vi "rename tag writer or reader.vi"(6 "new channel":refnum<class "TBM channel.lvclass">, 7 "owner ID":string, 8 "error in":errorcluster, 9 "old channel":refnum<class "TBM channel.lvclass">, 10 "tag descriptor":refnum<class "tag descriptor.lvclass">, 11 "engine configuration in":refnum<class "engine configuration.lvclass">) -> (0 "error out":errorcluster, 3 "engine configuration out":refnum<class "engine configuration.lvclass">)   [LabVIEW 2013, in "engine configuration.lvclass"]
uses:
  engine configuration.lvclass
  <vilib>/NI/Tag Bus/tag/tag descriptor.lvclass
  <vilib>/NI/Tag Bus Module Framework/channel/TBM channel.lvclass
  <vilib>/NI/Tag Bus/tag/tag descriptor.lvclass/tag descriptor.ctl
  engine configuration.lvclass/engine configuration.ctl
  <vilib>/NI/Tag Bus Module Framework/channel/TBM channel.lvclass/TBM channel.ctl
  <vilib>/NI/Tag Bus/tag/read tag name.vi
  <vilib>/NI/Tag Bus Module Framework/channel/Read channel classification.vi
  <vilib>/NI/Tag Bus Module Framework/root configuration/TBM configuration.lvclass
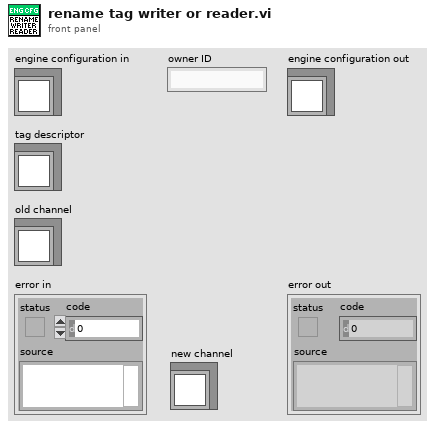
[diagram p1: front panel]
types:
  T1 = typedef "engine configuration.lvclass/Tag Info.ctl" = cluster{"Tag":refnum<class "tag descriptor.lvclass">, "Writer":string, "Readers":string[], "Owning ID":string}
  T2 = typedef "TBM channel.lvclass/channel classification.ctl" = enum16{"input data", "output data", "processing parameter", "processing result"}
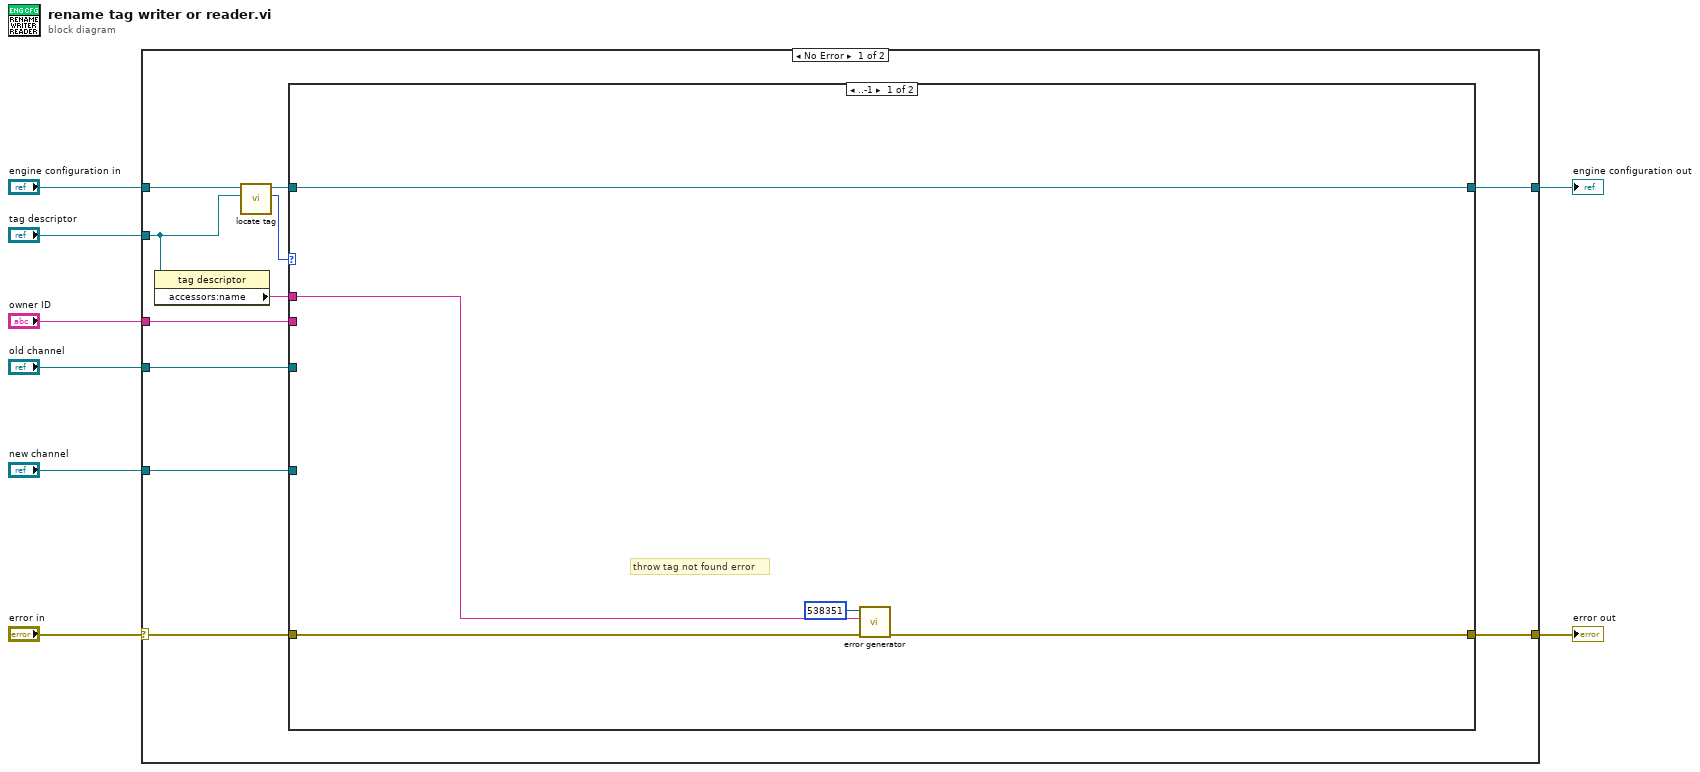
[diagram p0: block diagram]
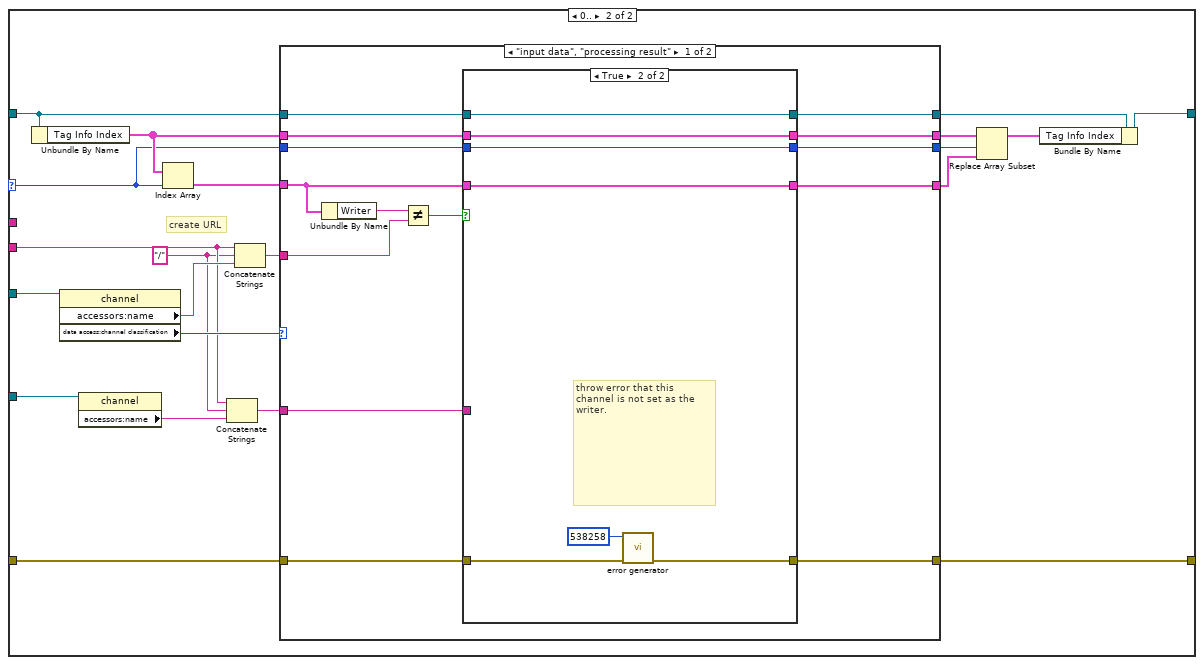
[diagram p2: hidden frame]
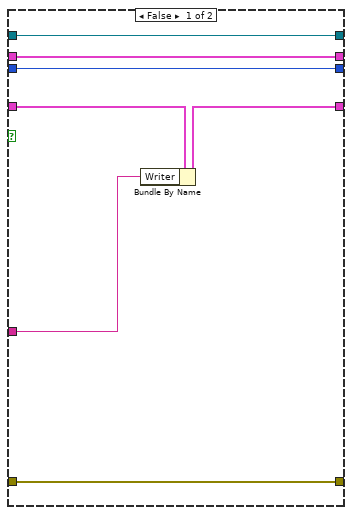
[diagram p3: hidden frame]
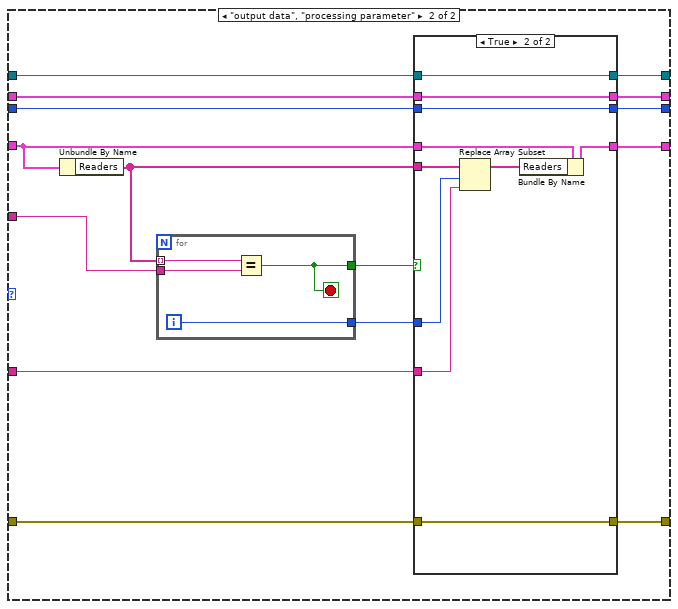
[diagram p4: hidden frame]
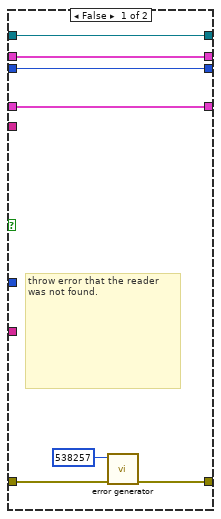
[diagram p5: hidden frame]
diagram:
  n1 = case shown="No Error" "error in" {
    selector: "error in" -> [w15 w111]
    tunnel: [w13 w111] -> w7
    tunnel: [w12 w110] -> w5
    tunnel: "engine configuration in" -> [w19 w110]
    tunnel: "tag descriptor" -> [w10 _]
    tunnel: "owner ID" -> [w16 _]
    tunnel: "old channel" -> [w17 _]
    tunnel: "new channel" -> [w11 _]
    frame No Error {
      n2 = property class="tag descriptor"(reference=w10) -> ("accessors:name"=w9:string)  [unwired: 1 in, 2 out]
      n3 = call "locate tag.vi"("tag descriptor"=w10, "engine configuration in"=w19) -> ("index"=w14:i32, "engine configuration out"=w18:refnum<class "engine configuration.lvclass">)  [unwired: 8 in]
      n4 = case shown="..-1" w14 {
        selector: w14 -> [_ w38]
        tunnel: w18 -> [w24 w37]
        tunnel: w17 -> [_ w45]
        tunnel: w16 -> [_ w28]
        tunnel: w15 -> [w22 w40]
        tunnel: [w21 w36] -> w13
        tunnel: [w24 w30] -> w12
        tunnel: w11 -> [_ w29]
        tunnel: w9 -> [w20 _]
        frame ..-1 {
          # "throw tag not found error"
          n5 = call <vilib>:"error generator.vi"("error in"=w22, "append error message"=w20, "error code (0)"=538351) -> ("error out"=w21:errorcluster)  [unwired: 8 in]
        }
        frame 0.. {
          w27 = "/" ("string")
          # "create URL"
          n6 = Unbundle By Name(w37) -> ("Tag Info Index"=w39:T1[])
          n7 = property class="channel"(reference=w45) -> ("accessors:name"=w44:string, "data access:channel classification"=w43:T2)  [unwired: 1 in, 2 out]
          n8 = property class="channel"(reference=w29) -> ("accessors:name"=w26:string)  [unwired: 1 in, 2 out]
          n9 = Index Array(array=w39, index=w38) -> (element=w41:T1)
          n10 = Concatenate Strings(w28, w27, w26) -> (w25:string)
          n11 = Concatenate Strings(w28, w27, w44) -> (w42:string)
          n12 = case shown="\"input data\", \"processing result\"" w43 {
            tunnel: w42 -> [w47 w86]
            tunnel: w41 -> [w56 w85]
            tunnel: w40 -> [w57 w81]
            tunnel: w39 -> [w51 w78]
            tunnel: w38 -> [w49 w76]
            tunnel: w37 -> [w54 w84]
            tunnel: [w53 w83] -> w32
            tunnel: [w55 w82] -> w33
            tunnel: [w52 w80] -> w36
            tunnel: [w50 w79] -> w34
            tunnel: [w48 w77] -> w35
            tunnel: w25 -> [w46 w74]
            frame "input data", "processing result" {
              n13 = Unbundle By Name(w56) -> ("Writer"=w59:string)
              n14 = Not Equal?(x=w59, y=w47) -> (x != y?=w58:bool)
              n15 = case shown="True" w58 {
                tunnel: w57 -> [w64 w68]
                tunnel: w56 -> [w66 w73]
                tunnel: [w65 w73] -> w55
                tunnel: [w64 w67] -> w52
                tunnel: w54 -> [w63 w72]
                tunnel: [w63 w72] -> w53
                tunnel: w51 -> [w62 w71]
                tunnel: [w62 w71] -> w50
                tunnel: w49 -> [w61 w70]
                tunnel: [w61 w70] -> w48
                tunnel: w46 -> [w60 _]
                frame False {
                  n16 = Bundle By Name(cluster=w66, "Writer"=w60) -> (w65:T1)
                }
                frame True {
                  # "throw error that this channel is not set as the writer."
                  n17 = call <vilib>:"error generator.vi"("error in"=w68, "error code (0)"=538258) -> ("error out"=w67:errorcluster)  [unwired: 9 in]
                }
              }
            }
            frame "output data", "processing parameter" {
              n18 = Unbundle By Name(w85) -> ("Readers"=w87:string[])
              n19 = for {
                tunnel: w87 -> [w108] mode=indexing
                tunnel: w86 -> [w109]
                tunnel: [w107] -> w88
                tunnel: [w106] -> w75
                i -> [w106]
                stop <- w107 stop-if-true
                n20 = Equal?(x=w108, y=w109) -> (x = y?=w107:bool)
              }
              n21 = case shown="True" w88 {
                tunnel: w87 -> [_ w99]
                tunnel: w85 -> [w94 w105]
                tunnel: w84 -> [w95 w104]
                tunnel: [w95 w104] -> w83
                tunnel: [w94 w103] -> w82
                tunnel: w81 -> [w90 w102]
                tunnel: [w89 w102] -> w80
                tunnel: [w93 w101] -> w79
                tunnel: w78 -> [w93 w101]
                tunnel: [w92 w100] -> w77
                tunnel: w76 -> [w92 w100]
                tunnel: w75 -> [_ w97]
                tunnel: w74 -> [_ w96]
                frame False {
                  # "throw error that the reader was not found."
                  n22 = call <vilib>:"error generator.vi"("error in"=w90, "error code (0)"=538257) -> ("error out"=w89:errorcluster)  [unwired: 9 in]
                }
                frame True {
                  n23 = Replace Array Subset(array=w99, new element=w96, index=w97) -> (w98:string[])
                  n24 = Bundle By Name(cluster=w105, "Readers"=w98) -> (w103:T1)
                }
              }
            }
          }
          n25 = Replace Array Subset(array=w34, new element=w33, index=w35) -> (w31:T1[])
          n26 = Bundle By Name(cluster=w32, "Tag Info Index"=w31) -> (w30:refnum<class "engine configuration.lvclass">)
        }
      }
    }
    frame Error {
    }
  }
  "error out" <- w7
  "engine configuration out" <- w5
